vi "Scope_5160_minimal.vi"() -> ()   [LabVIEW 2013]
uses:
  <vilib>/rvi/interface/nirviReadWriteControl/nirviReadWriteControl.xnode
  <vilib>/rvi/errors/niLvFpgaAdjustHostInterfaceError.vi
  <vilib>/rvi/interface/nirviCloseFPGA/nirviCloseFPGA.xnode
  NiFpgaLv.dll
  <vilib>/Utility/error.llb/Error Cluster From Error Code.vi
  <vilib>/rvi/interface/Simulation/niFpgaSimulationCallBeginRW.vi
  <vilib>/rvi/interface/nirviOpenFPGA/nirviOpenFPGA.xnode
  <vilib>/rvi/interface/nirviMethod/nirviMethod.xnode
  <resource>/objmgr/PeerToPeerStream.rc
  FPGA Bitfiles/mixer_FPGATarget_FPGA5160minimal_MG3sHgywKFM.lvbitx
  <vilib>/FPGAPlugInAG/Dynamic/niLvFpga_Close_Dynamic.vi
  <vilib>/FPGAPlugInAG/PXIe-7975R/niLvFpga_Open_PXIe-7975R.vi
  <vilib>/rvi/interface/common/dynamic/niFpgaDynamicAddResources.vi
  fpga_ref_minimal.ctl
  <vilib>/FPGAPlugInAG/Dynamic/niLvFpga_ReadFifo_Dynamic.vi
  <vilib>/rvi/errors/niLvFpgaMergeErrorWithErrorCode.vi
  <vilib>/userdefined/High Color/nirio_resource_hc.ctl
panel:
  in  "channel name":string="0,2"
  out "Writer:Overflow":bool
  out "Actual Sample Rate":dbl format="%#_6p"
  in  "min sample rate":dbl=97000000.0 format="%.2p"
  in  "SCOPE Resource":refnum<k15>="Dev1" caption="NI-Scope Resource"
  in  "Downsample rate":u32
  out "Timedata":i16[][](graph)
  in  "Acquire":bool
  in  "stop":bool
  in  "resource name":T1="RIO0"
  # "Set before running the VI"
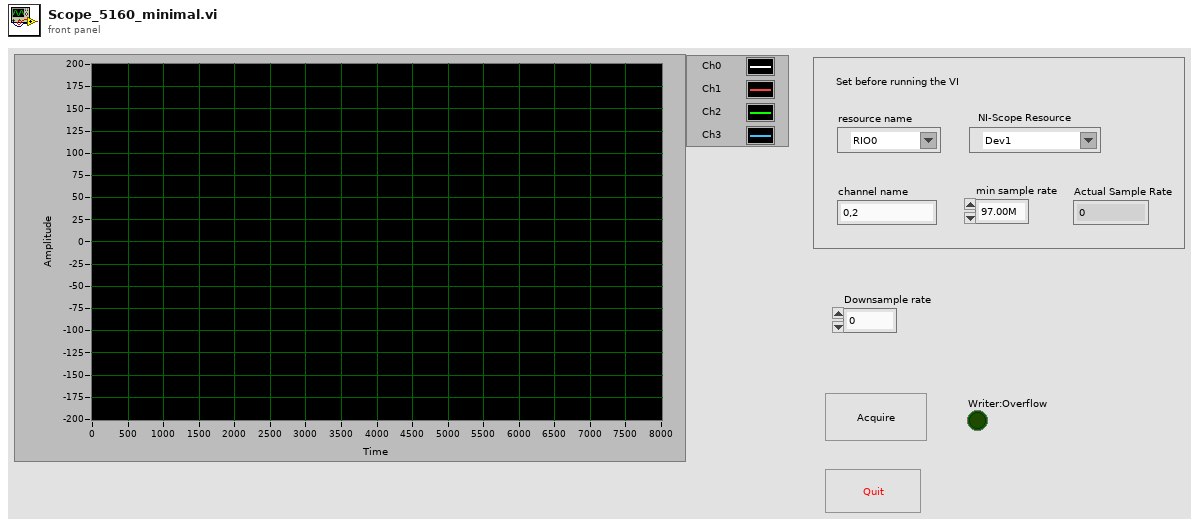
[diagram p1: front panel]
types:
  T1 = typedef "nirio_resource_hc.ctl" = tag
  T2 = typedef "5160FPGAref.ctl" = refnum<k20>
  T3 = typedef "fpga_ref_minimal.ctl" = refnum<k20>
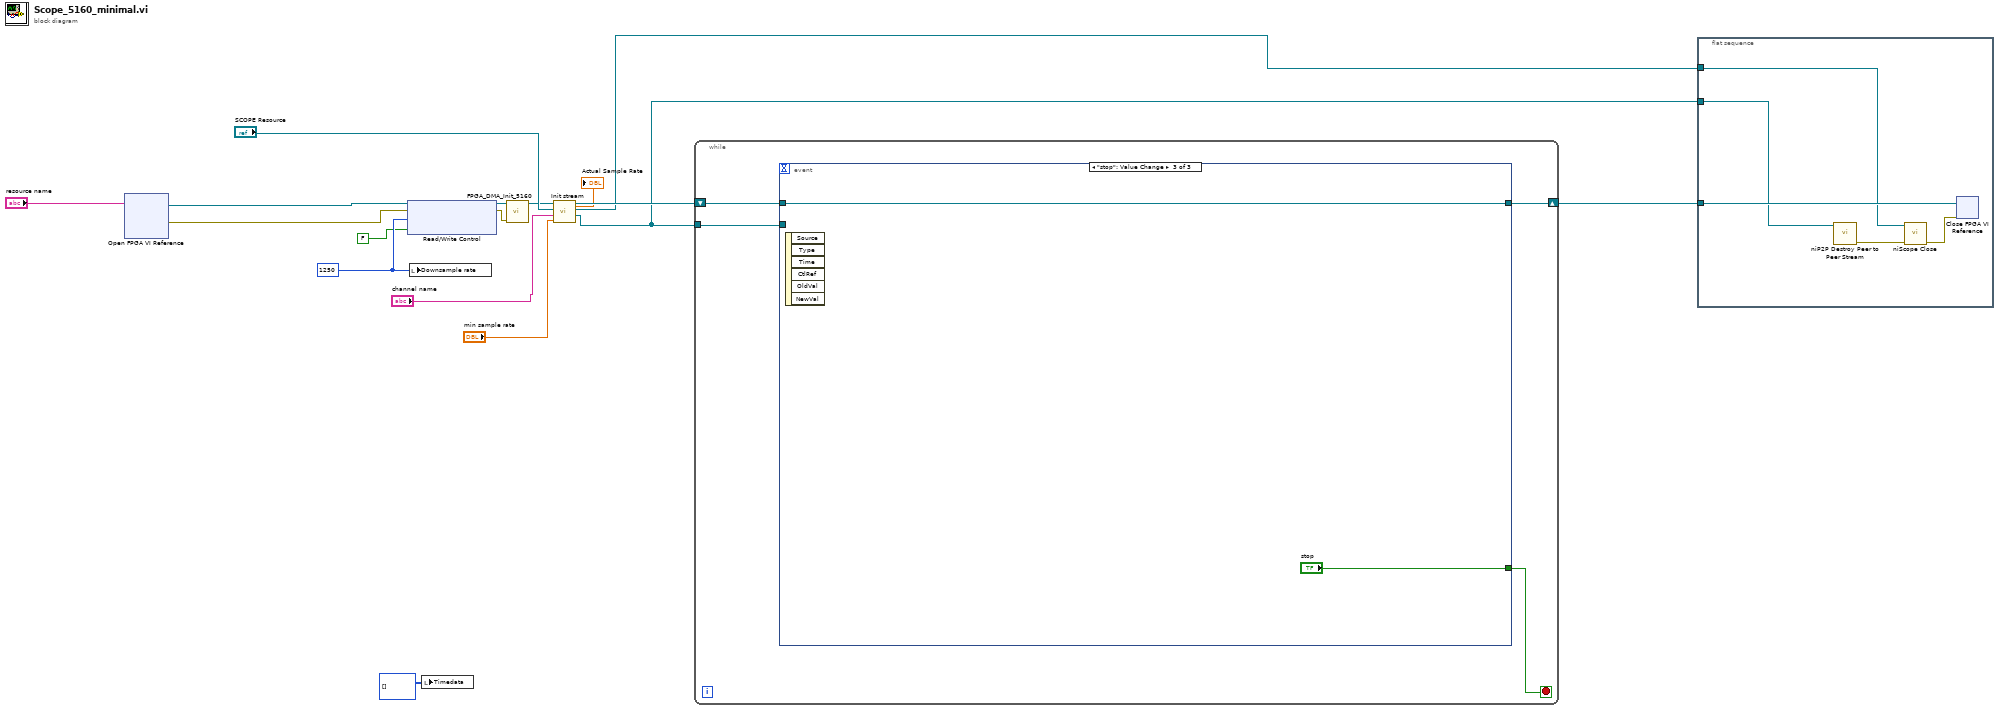
[diagram p0: block diagram]
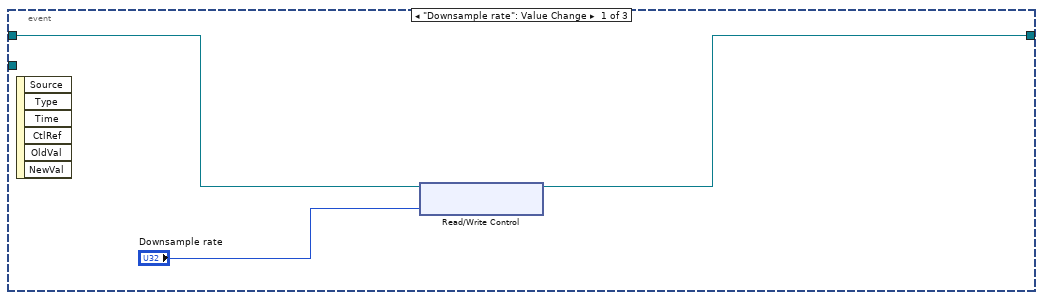
[diagram p2: hidden frame]
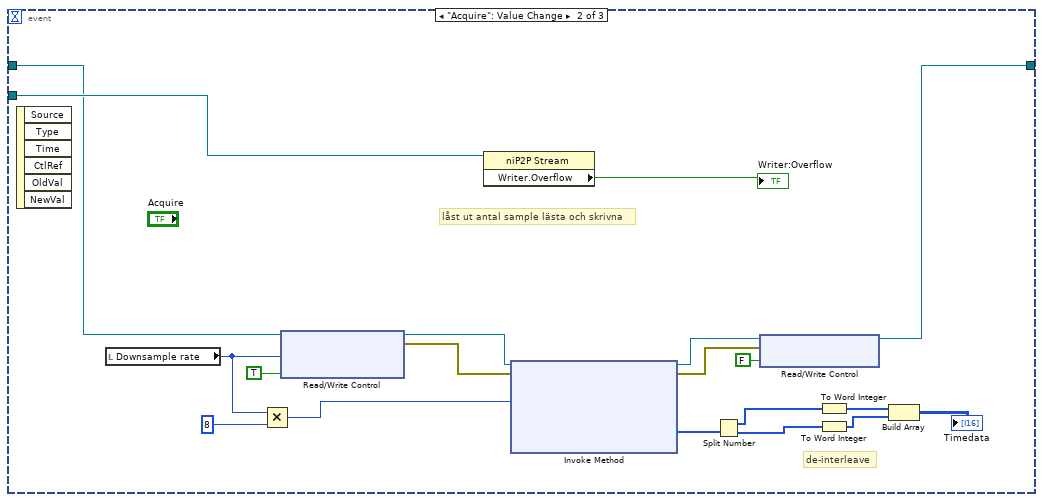
[diagram p3: hidden frame]
diagram:
  w17 = u32 1250 ("Samples to aqcuire")
  n1 = xnode "Open FPGA VI Reference"("resource name"="resource name") -> ("FPGA VI Reference Out"=w4:refnum<k20>, "error out"=w2:errorcluster)  [unwired: 1 in]
  n2 = xnode "Read/Write Control"("FPGA VI Reference In"=w4, "error in"=w2, "Samples Per Trigger"=w17, "Trigger Acquisition"=FALSE) -> ("FPGA VI Reference Out"=w5:refnum<k20>, "error out"=w6:errorcluster)
  n3 = local write "Downsample rate"(w17) -> ()
  n4 = local write "Timedata"(i16[][] [] ("Timedata")) -> ()
  n5 = call "FPGA_DMA_Init_5160.vi"("error in (no error)"=w6, "FPGA VI Reference"=w5) -> ("FPGA VI Reference 2"=w3:T2)  [unwired: 7 in, 2 out]
  n6 = call "Init stream.vi"("min sample rate"="min sample rate", "channel name"="channel name", "SCOPE Resource"="SCOPE Resource", "FPGA VI Reference"=w3) -> ("stream session"=w9:refnum<k20>, "instrument handle out"=w7:refnum<k15>, "FPGA VI Reference out"=w13:T3, "Actual Sample Rate"=→"Actual Sample Rate":dbl)  [unwired: 3 in, 1 out]
  n7 = while {
    shift-right: [w19] -> w12
    shift-left: w13 -> [w20]
    tunnel: w9 -> [w18]
    stop <- w21 stop-if-true
    n8 = event shown="[2] \"stop\": Value Change" {
      selector: _ -> [_ _ _]
      dyn-events: _ -> [_ _ _]
      timeout: _ -> [_ _ _]
      tunnel: [_ _ "stop"] -> w21
      tunnel: [w22 w33 w44] -> w19
      tunnel: w20 -> [w23 w25 w44]
      tunnel: w18 -> [_ w30 _]
      event "Downsample rate": Value Change {
        n9 = event-data() -> ()  [unwired: 1 in, 6 out]
        n10 = xnode "Read/Write Control"("FPGA VI Reference In"=w23, "Samples Per Trigger"="Downsample rate") -> ("FPGA VI Reference Out"=w22:T3)  [unwired: 1 in, 1 out]
      }
      event "Acquire": Value Change {
        # "låst ut antal sample lästa och skrivna"
        # "de-interleave"
        n11 = event-data() -> ()  [unwired: 1 in, 6 out]
        n12 = local read "Downsample rate"() -> (w34:u32)
        n13 = Multiply(x=w34, y=u32 8) -> (x*y=w38:u32)
        n14 = xnode "Read/Write Control"("FPGA VI Reference In"=w25, "Samples Per Trigger"=w34, "Trigger Acquisition"=TRUE) -> ("FPGA VI Reference Out"=w36:T3, "error out"=w41:errorcluster)  [unwired: 1 in]
        n15 = property class="niP2P Stream"(reference=w30) -> ("Writer.Overflow"=→"Writer:Overflow":bool)  [unwired: 1 in, 2 out]
        n16 = xnode "Invoke Method"("FPGA VI Reference In"=w36, "error in"=w41, "Number of Elements"=w38) -> ("FPGA VI Reference Out"=w42:T3, "error out"=w40:errorcluster, "Data"=w28:u32[])  [unwired: 1 in, 1 out]
        n17 = Split Number(x=w28) -> (hi(x)=w27:u16[], lo(x)=w26:u16[])
        n18 = xnode "Read/Write Control"("FPGA VI Reference In"=w42, "error in"=w40, "Trigger Acquisition"=FALSE) -> ("FPGA VI Reference Out"=w33:T3)  [unwired: 1 out]
        n19 = To Word Integer(number=w27) -> (16bit integer=w37:i16[])
        n20 = To Word Integer(number=w26) -> (16bit integer=w31:i16[])
        n21 = Build Array(w37, w31) -> (→"Timedata":i16[][])
      }
      event "stop": Value Change {
        n22 = event-data() -> ()  [unwired: 1 in, 6 out]
      }
    }
  }
  n23 = flat-sequence {
    tunnel: w12 -> [w48]
    tunnel: w7 -> [w47]
    tunnel: w9 -> [w46]
    frame #0 {
      n24 = call <vilib>:"niP2P Destroy Peer to Peer Stream.vi"("stream session"=w46) -> ("error out"=w50:errorcluster)  [unwired: 14 in]
      n25 = call <instrlib>:"niScope Close.vi"("instrument handle"=w47, "error in"=w50) -> ("error out"=w49:errorcluster)  [unwired: 13 in]
      n26 = xnode "Close FPGA VI Reference"("FPGA VI Reference In"=w48, "error in"=w49) -> ()  [unwired: 1 out]
    }
  }
